vi "iWorx Light & Laser SubVI (Periodic).vi"(7 "# of Timestamps to store (10)":u32=10, 9 "Threshold":dbl, 11 "Waveform":waveform(dbl)) -> (0 "Falling Edge Times":timestamp[](array[timestamp]), 1 "Rising Edge Times":timestamp[](array[timestamp]), 2 "Beam Break Durration (s)":dbl[](array[numeric]), 3 "Rising Edge Delta t (s)":dbl[](array[numeric]))   [LabVIEW 2012]
doc: "This sub VI takes a single <b> Waveform</b> input from the iWorx Light & Laser sensor. It returns timing data for periodic events The <b>Rising Edge Delta t</b> array gives the difference in time between each succesive rising edge in seconds. The <b>Beam Break Durations </b> is how long the laser was blocked for so you calculate speed based the width of an object."
uses:
  <vilib>/ptbypt/NI_PtbyPt.lvlib
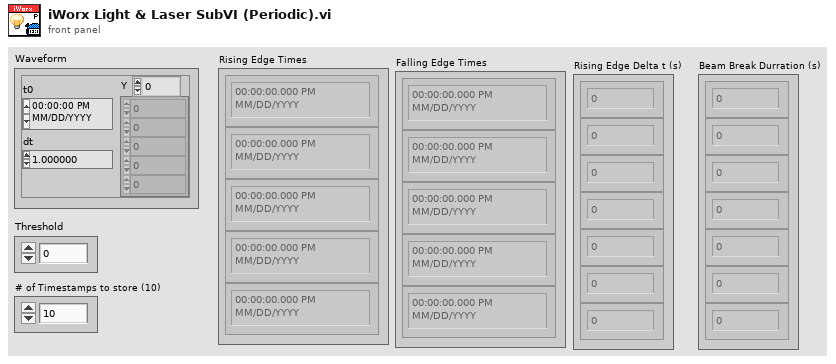
[diagram p1: front panel]
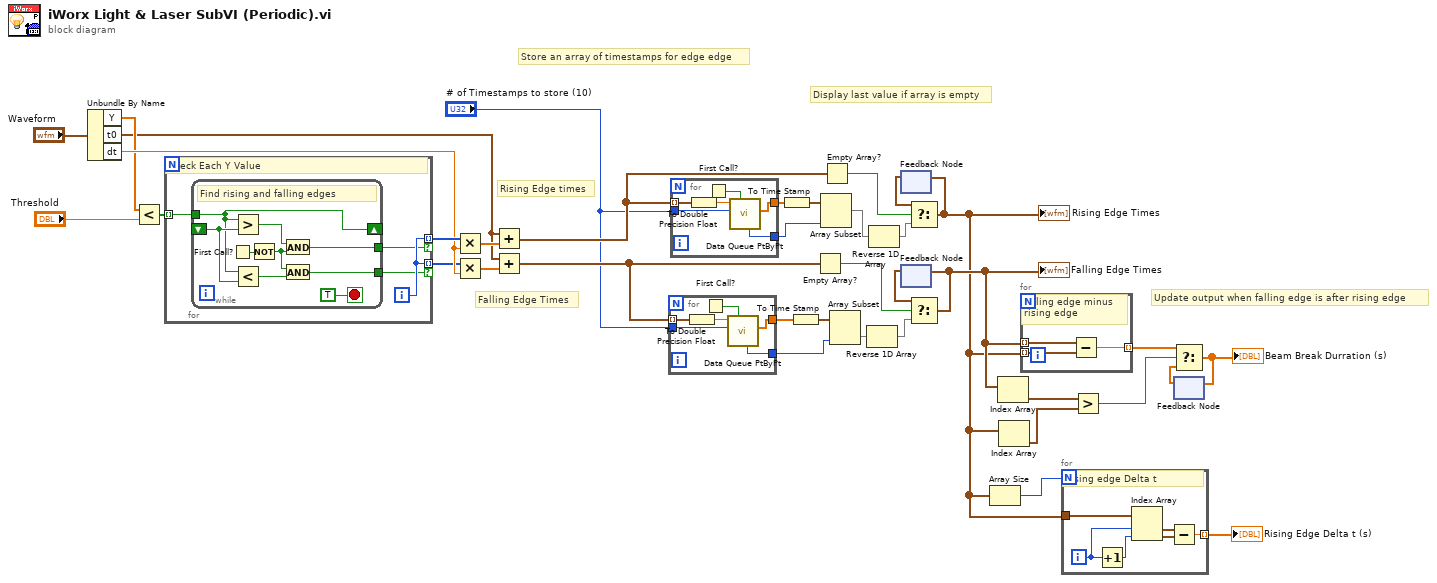
[diagram p0: block diagram]
diagram:
  # "Update output when falling edge is after rising edge"
  # "Store an array of timestamps for edge edge"
  # "Display last value if array is empty"
  # "Falling Edge Times"
  # "Rising Edge times"
  n1 = Unbundle By Name("Waveform") -> ("Y"=w32:dbl[], "t0"=w29:timestamp, "dt"=w34:dbl)
  n2 = Less?(x=w32, y="Threshold") -> (x < y?=w31:bool[])
  n3 = for {
    tunnel: [w41] -> w33 mode=indexing if=w39
    tunnel: [w41] -> w35 mode=indexing if=w38
    tunnel: w31 -> [w40] mode=indexing
    i -> [w41]
    # "Check Each Y Value"
    n4 = while {
      shift-right: [w44] -> _
      shift-left: _ -> [w49]
      tunnel: w40 -> [w44]
      tunnel: [w43] -> w39
      tunnel: [w42] -> w38
      stop <- TRUE stop-if-true
      # "Find rising and falling edges"
      n5 = First Call?() -> (First Call?: T/F=w45:bool)
      n6 = Greater?(x=w44, y=w49) -> (0:w50:bool)
      n7 = Less?(x=w44, y=w49) -> (x < y?=w48:bool)
      n8 = Not(x=w45) -> (.not. x?=w46:bool)
      n9 = And(x=w50, y=w46) -> (x .and. y?=w42:bool)
      n10 = And(x=w46, y=w48) -> (x .and. y?=w43:bool)
    }
  }
  n11 = Multiply(x=w35, y=w34) -> (x*y=w30:dbl[])
  n12 = Multiply(x=w33, y=w34) -> (x*y=w28:dbl[])
  n13 = Add(x=w29, y=w30) -> (x+y=w11:timestamp[])
  n14 = Add(x=w29, y=w28) -> (x+y=w23:timestamp[])
  n15 = for {
    tunnel: w23 -> [w56] mode=indexing
    tunnel: "# of Timestamps to store (10)" -> [w54]
    tunnel: [w53] -> w12
    tunnel: [w52] -> w6
    n16 = To Double Precision Float(number=w56) -> (double precision float=w55:dbl)
    n17 = First Call?() -> (First Call?: T/F=w51:bool)
    n18 = call <vilib>:"Data Queue PtByPt.vi"("initialize"=w51, "sample length"=w54, "input data point"=w55) -> ("Current Queue"=w52:dbl[], "current length"=w53:i32)  [unwired: 4 in, 3 out]
  }
  n19 = for {
    tunnel: w11 -> [w62] mode=indexing
    tunnel: "# of Timestamps to store (10)" -> [w60]
    tunnel: [w59] -> w8
    tunnel: [w58] -> w7
    n20 = To Double Precision Float(number=w62) -> (double precision float=w61:dbl)
    n21 = First Call?() -> (First Call?: T/F=w57:bool)
    n22 = call <vilib>:"Data Queue PtByPt.vi"("initialize"=w57, "sample length"=w60, "input data point"=w61) -> ("Current Queue"=w58:dbl[], "current length"=w59:i32)  [unwired: 4 in, 3 out]
  }
  n23 = To Time Stamp(1:w7) -> (0:w9:timestamp[])
  n24 = To Time Stamp(1:w6) -> (0:w13:timestamp[])
  n25 = Empty Array?(array=w23) -> (empty?=w22:bool)
  n26 = Array Subset(array=w9, length=w8) -> (w3:timestamp[])  [unwired: 1 in]
  n27 = Empty Array?(array=w11) -> (empty?=w24:bool)
  n28 = Array Subset(array=w13, length=w12) -> (w5:timestamp[])  [unwired: 1 in]
  n29 = Reverse 1D Array(array=w5) -> (reversed array=w4:timestamp[])
  n30 = Reverse 1D Array(array=w3) -> (reversed array=w2:timestamp[])
  n31 = feedback #1() -> (w37:timestamp[])  [unwired: 1 in]
  n32 = feedback #2() -> (w36:timestamp[])  [unwired: 1 in]
  n33 = Select(t=w37, s=w24, f=w2) -> (s? t:f=w16:timestamp[])
  "Rising Edge Times" <- w16
  n34 = feedback-in #1(w16) -> ()
  n35 = Select(t=w36, s=w22, f=w4) -> (s? t:f=w17:timestamp[])
  "Falling Edge Times" <- w17
  n36 = feedback-in #2(w17) -> ()
  n37 = Array Size(array=w16) -> (size(s)=w1:i32)
  n38 = Index Array(array=w17) -> (element=w21:timestamp)  [unwired: 1 in]
  n39 = Index Array(array=w16) -> (element=w20:timestamp)  [unwired: 1 in]
  n40 = for {
    tunnel: w16 -> [w64] mode=indexing
    tunnel: w17 -> [w65] mode=indexing
    tunnel: [w63] -> w19 mode=indexing
    # "falling edge minus  rising edge"
    n41 = Subtract(x=w65, y=w64) -> (x-y=w63:dbl)
  }
  n42 = for {
    N: w1 -> [_]
    tunnel: w16 -> [w71]
    tunnel: [w66] -> w14 mode=indexing
    i -> [w70]
    # "Rising edge Delta t"
    n43 = Increment(x=w70) -> (x+1=w69:i32)
    n44 = Index Array(array=w71, index #1=w70, index #2=w69) -> (element #1=w68:timestamp, element #2=w67:timestamp)
    n45 = Subtract(x=w68, y=w67) -> (x-y=w66:dbl)
  }
  "Rising Edge Delta t (s)" <- w14
  n46 = Greater?(x=w21, y=w20) -> (0:w18:bool)
  n47 = feedback #3() -> (w27:dbl[])  [unwired: 1 in]
  n48 = Select(t=w19, s=w18, f=w27) -> (s? t:f=w15:dbl[])
  "Beam Break Durration (s)" <- w15
  n49 = feedback-in #3(w15) -> ()
